vi "Convert Signals to Frame by ID.vi"(8 "error in (no error)":errorcluster, 9 "ID":u32, 10 "Data Ref":T2, 11 "Scale Ref":T3) -> (0 "error out":errorcluster, 2 "Found?":bool, 3 "Frame":T1 {"Identifier" format="%08x"})   [LabVIEW 2013, in "J1939 Addon Engine.lvlib"]
uses:
  J1939 Addon Engine.lvlib
  Types/Conversion Lookup Table Reference.ctl
  Types/Data Lookup Table Reference.ctl
  Types/Datatable Lookup DVR.ctl
  Shared/J1939 Utilities/Types/CAN Outgoing Message Cluster.ctl
  Conversion Lookup Table.vi
  <vilib>/xnet/xnet.llb/XNET Convert (Signal to Frame Raw).vi
  Data Lookup Table.vi
  Shared/J1939 Utilities/J1939 Utilities.lvlib
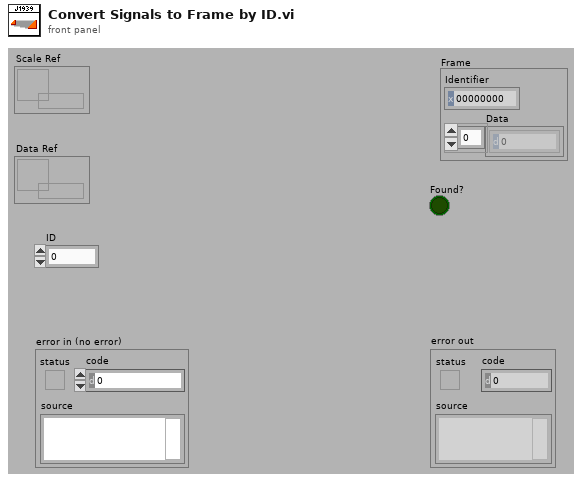
[diagram p1: front panel]
types:
  T1 = typedef "J1939 Addon Shared.lvlib/J1939 Utilities.lvlib/CAN Outgoing Message Cluster.ctl" = cluster{"Identifier":u32, "Data":u8[]}
  T2 = typedef "J1939 Addon Engine.lvlib/Data Lookup Table Reference.ctl" = refnum<data-value>
  T3 = typedef "J1939 Addon Engine.lvlib/Conversion Lookup Table Reference.ctl" = refnum<data-value>
  T4 = typedef "J1939 Addon Engine.lvlib/Conversion Lookup Table Parameters Cluster.ctl" = cluster{"Conversion":refnum<k21>, "Array Position":cluster{"Offset":u32, "Length":u32}, "Length":u32, "Conv ID":u32}
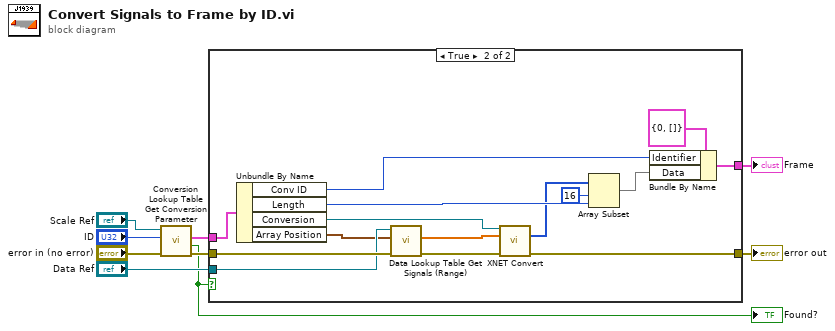
[diagram p0: block diagram]
diagram:
  n1 = call "Conversion Lookup Table Get Conversion Parameter.vi"("error in (no error)"="error in (no error)", "ID"="ID", "Scale Ref"="Scale Ref") -> ("error out"=w8:errorcluster, "Found?"=w1:bool, "Parameters"=w9:T4)  [unwired: 5 in, 1 out]
  "Found?" <- w1
  n2 = case shown="True" w1 {
    tunnel: w9 -> [_ w25]
    tunnel: w8 -> [w10 w24]
    tunnel: [w10 w20] -> w7
    tunnel: "Data Ref" -> [_ w19]
    tunnel: [_ w17] -> w3
    frame False {
    }
    frame True {
      n3 = Unbundle By Name(w25) -> ("Conv ID"=w11:u32, "Length"=w14:u32, "Conversion"=w16:refnum<k21>, "Array Position"=w15:cluster{"Offset":u32, "Length":u32})
      n4 = call "Data Lookup Table Get Signals (Range).vi"("error in (no error)"=w24, "Direct Access"=w15, "Data Ref"=w19) -> ("error out"=w23:errorcluster, "Signals"=w13:dbl[])  [unwired: 6 in, 1 out]
      n5 = call-poly <vilib>:"XNET Convert.vi"("session in"=w16, "signal data"=w13, "error in (no error)"=w23) -> ("frame data"=w12:u8[], "error out"=w20:errorcluster)  [unwired: 10 in, 1 out]
      n6 = Array Subset(array=w12, index=16, length=w14) -> (w21:u8[])
      n7 = Bundle By Name(cluster=T1 {"Identifier"=0, "Data"=[]} ("element"), "Identifier"=w11, "Data"=w21) -> (w17:T1)
    }
  }
  "error out" <- w7
  "Frame" <- w3
